vi "Load Async.vi"(7 "Deck ID":string, 8 "error in (no error)":errorcluster, 9 "Message Queue":refnum<queue>, 10 "Path":path, 11 "Audio Data Reference":refnum<data-value>) -> (0 "error out":errorcluster)   [LabVIEW 2018, in "Audio File Input.lvlib"]
doc: "This VI loads an audio track, placing the audio data into the specified DVR.\n\n<b>Priority:</b> Background\n<b>Execution System:</b> Other 1"
uses:
  Audio File Input.lvlib
  Messaging/Message Cluster.ctl
  Audio File Info.ctl
  <vilib>/Analysis/5stat.llb/RMS (DBL).vi
  Globals/Constants.vi
  <vilib>/measure/maresamp.llb/Resample N Waveforms (single shot).vi
  Messaging/Messaging.lvlib
  <vilib>/Analysis/NI_AALPro.lvlib
  Audio Processing/Audio Processing.lvlib
  Globals/Globals.lvlib
  <vilib>/measure/NI_MAPro.lvlib
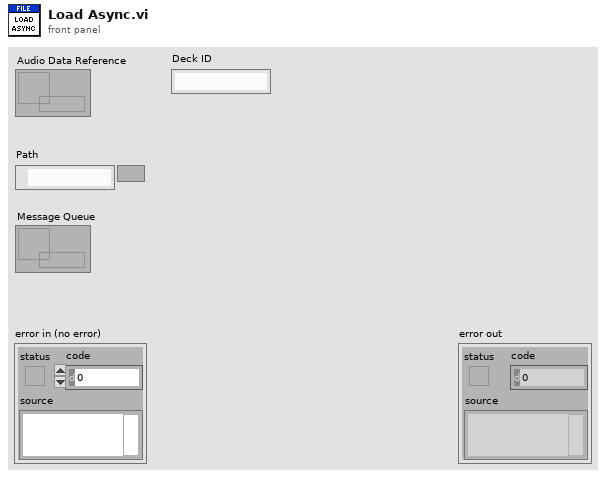
[diagram p1: front panel]
types:
  T1 = typedef "Messaging.lvlib/Message Cluster.ctl" = cluster{"Event":string, "Source":string, "Target":string, "Data":variant}
  T2 = typedef "Audio File Input.lvlib/Audio File Info.ctl" = cluster{"Length (Samples)":i32, "Channels":i32, "Sample Rate (Hz)":i32, "Path":path, "BPM":dbl, "Cue Points (Samples)":i32[]}
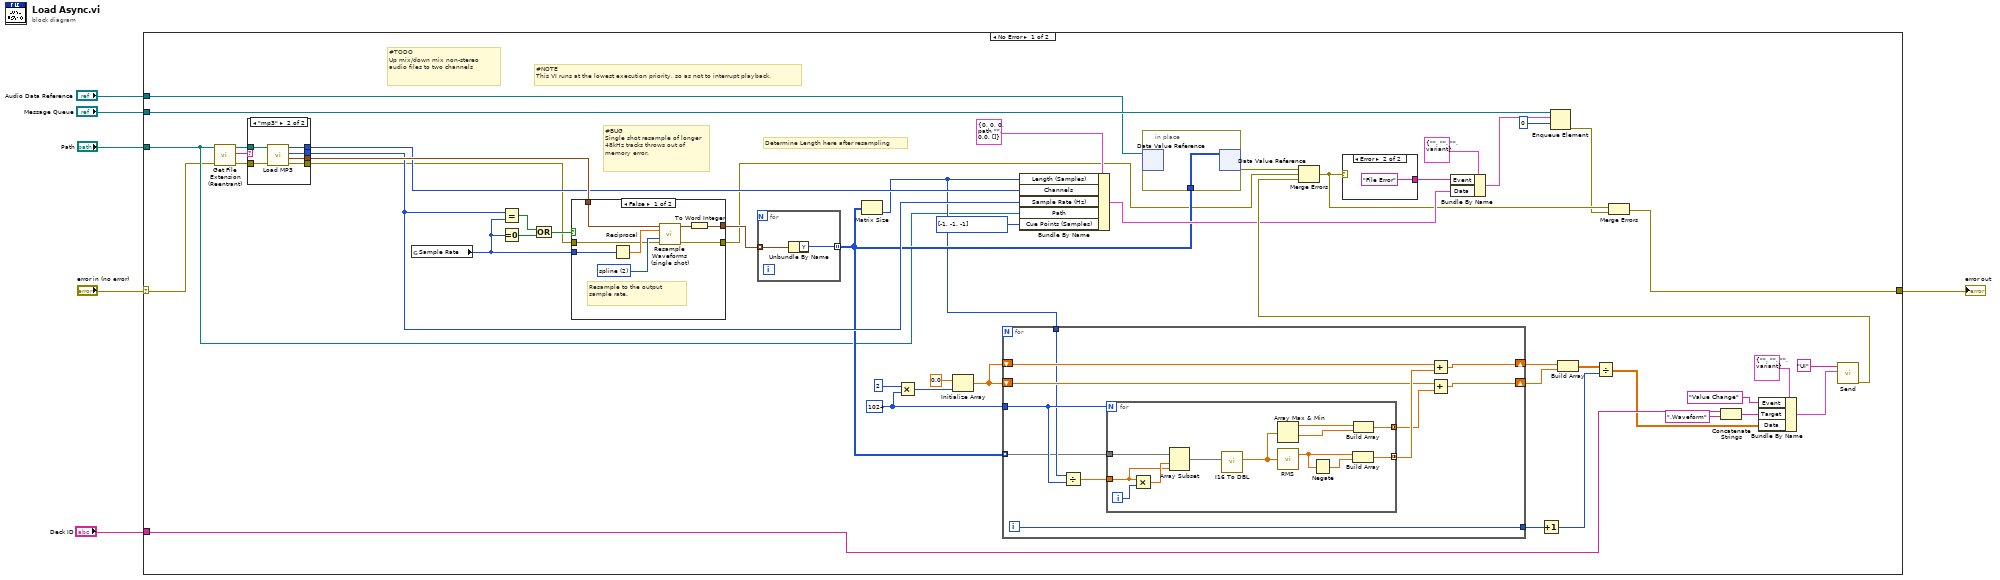
[diagram p0: block diagram]
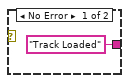
[diagram p2: hidden frame]
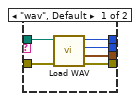
[diagram p3: hidden frame]
diagram:
  n1 = case shown="No Error" "error in (no error)" {
    selector: "error in (no error)" -> [w15 w106]
    tunnel: [w9 w106] -> w5
    tunnel: "Path" -> [w16 _]
    tunnel: "Message Queue" -> [w52 _]
    tunnel: "Audio Data Reference" -> [w46 _]
    tunnel: "Deck ID" -> [w33 _]
    frame No Error {
      w44 = 1024 ("y")
      # "#BUG\nSingle shot resample of longer 48kHz tracks throws out of memory error."
      # "Determine Length here after resampling"
      # "#TODO\nUp mix/down mix non-stereo audio files to two channels"
      # "#NOTE\nThis VI runs at the lowest execution priority, so as not to interrupt playback."
      n2 = call "Get File Extension (Reentrant).vi"("error in (no error)"=w15, "file"=w16) -> ("error out"=w14:errorcluster, "lowercase file extension"=w13:string, "dup file"=w12:path)  [unwired: 5 in, 2 out]
      n3 = case shown="\"mp3\"" w13 {
        tunnel: w12 -> [w62 w69]
        tunnel: w14 -> [w63 w68]
        tunnel: [w58 w67] -> w8
        tunnel: [w59 w66] -> w24
        tunnel: [w61 w65] -> w23
        tunnel: [w60 w64] -> w22
        frame "wav", Default {
          n4 = call "Load WAV.vi"("error in (no error)"=w63, "Path"=w62) -> ("error out"=w58:errorcluster, "data"=w59:waveform(i16)[], "Sample Rate (Hz)"=w60:i32, "Channels"=w61:i32)  [unwired: 5 in, 1 out]
        }
        frame "mp3" {
          n5 = call "Load MP3.vi"("error in (no error)"=w68, "Path"=w69) -> ("error out"=w67:errorcluster, "data"=w66:waveform(i16)[], "Sample Rate (Hz)"=w64:i32, "Channels"=w65:i32)  [unwired: 5 in, 1 out]
        }
      }
      n6 = global read "Constants.vi" "Sample Rate"() -> (w17:i32)
      n7 = Equal?(x=w22, y=w17) -> (x = y?=w55:bool)
      n8 = Equal To 0?(x=w17) -> (x = 0?=w54:bool)
      n9 = Or(x=w55, y=w54) -> (x .or. y?=w53:bool)
      n10 = case shown="False" w53 {
        tunnel: w24 -> [w100 w105]
        tunnel: w17 -> [w102 _]
        tunnel: [w98 w105] -> w50
        tunnel: w8 -> [w97 w104]
        tunnel: [w96 w104] -> w7
        frame False {
          w103 = u16 2 items=["coerce", "linear", "spline", "FIR filter"] ("interpolation mode")
          # "Resample to the output sample rate."
          n11 = Reciprocal(x=w102) -> (1/x=w101:dbl)
          n12 = call-poly <vilib>:"Resample Waveforms (single shot).vi"("waveforms in"=w100, "dt"=w101, "interpolation mode"=w103, "error in (no error)"=w97) -> ("resampled waveforms out"=w99:waveform(dbl)[], "error out"=w96:errorcluster)  [unwired: 8 in, 2 out]
          n13 = To Word Integer(number=w99) -> (16bit integer=w98:waveform(i16)[])
        }
        frame True {
        }
      }
      n14 = for {
        tunnel: w50 -> [w95] mode=indexing
        tunnel: [w94] -> w19 mode=indexing
        n15 = Unbundle By Name(w95) -> ("Y"=w94:i16[])
      }
      n16 = Matrix Size(0:w19) -> (2:w18:i32)  [unwired: 1 out]
      n17 = Multiply(x=2, y=w44) -> (x*y=w37:i32)
      n18 = Initialize Array(0.0 ("element"), w37) -> (w41:dbl[])
      n19 = for {
        tunnel: w19 -> [w71] mode=indexing
        tunnel: w44 -> [w80]
        shift-right: [w75] -> w40
        shift-left: w41 -> [w78]
        shift-right: [w74] -> w39
        shift-left: w41 -> [w77]
        tunnel: w18 -> [w72]
        tunnel: [w70] -> w36
        i -> [w70]
        n20 = Divide(x=w72, y=w80) -> (x/y=w73:dbl)
        n21 = for {
          N: w80 -> [_]
          tunnel: w71 -> [w92]
          tunnel: [w85] -> w76 mode=concatenating
          tunnel: [w84] -> w79 mode=concatenating
          tunnel: w73 -> [w83]
          i -> [w91]
          n22 = Multiply(x=w83, y=w91) -> (x*y=w90:dbl)
          n23 = Array Subset(array=w92, index=w90, length=w83) -> (w82:i16[])
          n24 = call "I16 To DBL.vi"("Audio Data (1D I16)"=w82) -> ("Audio Data (1D DBL)"=w81:dbl[])  [unwired: 9 in, 1 out]
          n25 = Array Max & Min(array=w81) -> (max value=w87:dbl, min value=w86:dbl)  [unwired: 2 out]
          n26 = call-poly <vilib>:"RMS.vi"("X"=w81) -> ("rms value"=w89:dbl)  [unwired: 1 out]
          n27 = Negate(x=w89) -> (-x=w88:dbl)
          n28 = Build Array(w89, w88) -> (w84:dbl[])
          n29 = Build Array(w87, w86) -> (w85:dbl[])
        }
        n30 = Add(x=w78, y=w79) -> (x+y=w75:dbl[])
        n31 = Add(x=w77, y=w76) -> (x+y=w74:dbl[])
      }
      n32 = Bundle By Name(cluster=T2 {"Length (Samples)"=0, "Channels"=0, "Sample Rate (Hz)"=0, "Path"=path "", "BPM"=0.0, "Cue Points (Samples)"=[]} ("Track Info"), "Length (Samples)"=w18, "Channels"=w23, "Sample Rate (Hz)"=w22, "Path"=w16, "Cue Points (Samples)"=i32[] [-1, -1, -1]) -> (w21:T2)
      n33 = in-place {
        in-place-border: w19 -> [w93]
        n34 = in-place-dvr #1(w46) -> ()  [unwired: 2 out]
        n35 = in-place-dvr #1(w93) -> (w45:errorcluster)  [unwired: 1 out]
      }
      n36 = Increment(x=w36) -> (x+1=w35:i32)
      n37 = Build Array(w40, w39) -> (w38:dbl[][])
      n38 = Divide(x=w38, y=w35) -> (x/y=w26:dbl[][])
      n39 = Concatenate Strings(w33, ".Waveform" ("string")) -> (w30:string)
      n40 = Bundle By Name(cluster=T1 {"Event"="", "Source"="", "Target"="", "Data"=variant} ("Message"), "Event"="Value Change", "Target"=w30, "Data"=w26) -> (w27:T1)
      n41 = call "Send.vi"("Message"=w27, "Queue Name"="UI") -> ("error out"=w25:errorcluster)  [unwired: 9 in]
      n42 = Merge Errors(w45, w7, w25) -> (w11:errorcluster)
      n43 = case shown="Error" w11 {
        tunnel: ["Track Loaded" ("Type") "File Error" ("Type")] -> w47
        frame No Error {
        }
        frame Error {
        }
      }
      n44 = Bundle By Name(cluster=T1 {"Event"="", "Source"="", "Target"="", "Data"=variant} ("element"), "Event"=w47, "Data"=w21) -> (w48:T1)
      n45 = Enqueue Element(queue=w52, element=w48, timeout in ms (-1)=0) -> (error out=w10:errorcluster)  [unwired: 1 in, 2 out]
      n46 = Merge Errors(w11, w10) -> (w9:errorcluster)
    }
    frame Error {
    }
  }
  "error out" <- w5
